vi "UDP ROS Reciever.vi"(8 "error in (no error)":errorcluster, 9 "ENQUE DIRECTLY":refnum<queue>, 10 "milliseconds to wait":u32, 11 "UDP Network Connection in":refnum<k16>) -> (0 "error out":errorcluster)   [LabVIEW 2016]
uses:
  Globale Variable/Globale Variable.vi
panel:
  out "data out":string
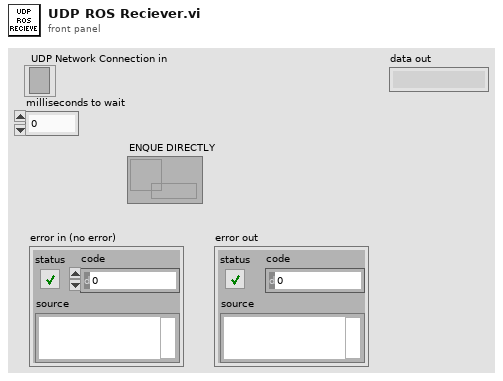
[diagram p1: front panel]
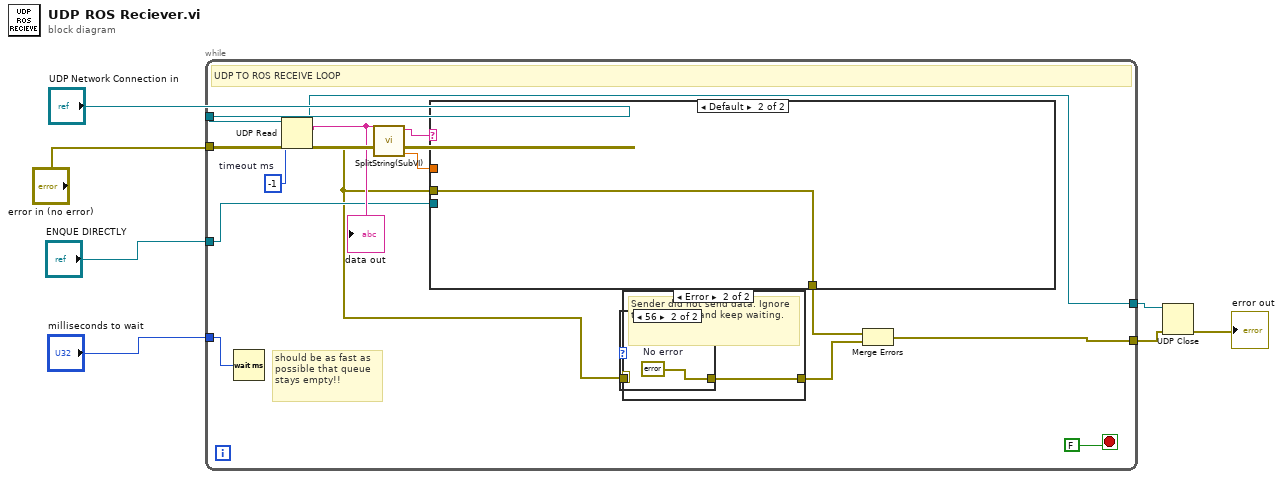
[diagram p0: block diagram]
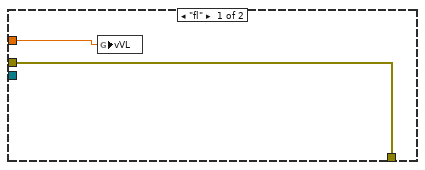
[diagram p2: hidden frame]
diagram:
  n1 = while {
    tunnel: [w18] -> w6
    tunnel: "UDP Network Connection in" -> [w20]
    tunnel: "error in (no error)" -> [w19]
    tunnel: "milliseconds to wait" -> [w14]
    tunnel: [w11] -> w2
    tunnel: "ENQUE DIRECTLY" -> [w10]
    stop <- FALSE stop-if-true
    w21 = -1  # timeout ms
    # "should be as fast as possible that queue stays empty!!"
    # "UDP TO ROS RECEIVE LOOP"
    n2 = Wait (ms)(milliseconds to wait=w14) -> ()  [unwired: 1 out]
    n3 = UDP Read(connection ID=w20, timeout ms (25000)=w21, 8:w19) -> (data out=w15:string, error out=w9:errorcluster, 3:w18:refnum<k16>)  [unwired: 3 out]
    "data out" <- w15
    n4 = call "SplitString(SubVI).vi"("data in"=w15) -> ("Numeric"=w17:dbl, "String 3"=w16:string)  [unwired: 9 in]
    n5 = case shown="Default" w16 {
      tunnel: w17 -> [w22 _]
      tunnel: w9 -> [w23 w24]
      tunnel: [w23 w24] -> w12
      tunnel: w10 -> [_ _]
      frame "fl" {
        n6 = global write "Globale Variable.vi" "vVL"(w22) -> ()
      }
      frame Default {
      }
    }
    n7 = case shown="Error" w9 {
      selector: w9 -> [w25 w27]
      tunnel: [w25 w26] -> w13
      frame No Error {
        # "Sender sent data. Update the chart value."
      }
      frame Error {
        # "Sender did not send data. Ignore timeout error and keep waiting."
        n8 = Unbundle By Name(w27) -> ("code"=w28:i32)
        n9 = case shown="56" w28 {
          tunnel: w27 -> [w29 _]
          tunnel: [w29 w30] -> w26
          frame Default {
          }
          frame 56 {
            w30 = errorcluster {"status"=FALSE, "code"=0, "source"=""}  # No error
          }
        }
      }
    }
    n10 = Merge Errors(w12, w13) -> (w11:errorcluster)
  }
  n11 = UDP Close(connection ID=w6, 8:w2) -> (error out=→"error out":errorcluster)  [unwired: 1 out]
